vi "RSZVB Get All Calibration Units.vi"(8 "error in (no error)":errorcluster {"code" format="%.0x"}, 11 "VISA session":refnum<visa-resource-name>) -> (0 "error out":errorcluster {"code" format="%.0x"}, 2 "Calibration Unit":string, 3 "dup VISA session":refnum<visa-resource-name>)   [LabVIEW 2011]
doc: "This VI returns the type and address of all calibration units connected to the VNA. \n\nRemote-control command(s):\n:SYSTem:COMMunicate:RDEVice:AKAL:ADDRess:ALL?"
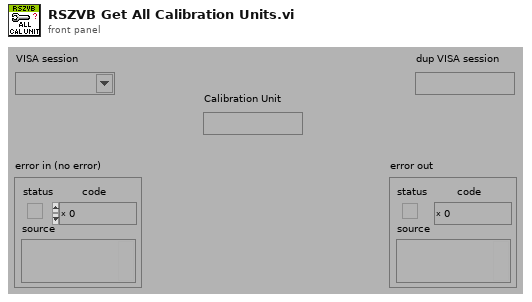
[diagram p1: front panel]
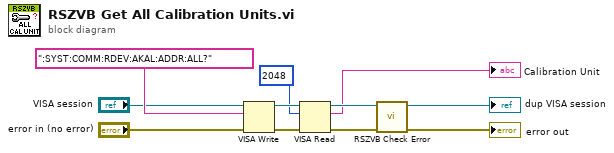
[diagram p0: block diagram]
diagram:
  n1 = VISA Write(VISA resource name="VISA session", write buffer=":SYST:COMM:RDEV:AKAL:ADDR:ALL?" ("format string"), error in (no error)="error in (no error)") -> (VISA resource name out=w10:refnum<visa-resource-name>, error out=w9:errorcluster)  [unwired: 1 out]
  n2 = VISA Read(VISA resource name=w10, byte count=u32 2048 ("byte count (0)"), error in (no error)=w9) -> (VISA resource name out=w7:refnum<visa-resource-name>, read buffer=→"Calibration Unit":string, error out=w6:errorcluster)  [unwired: 1 out]
  n3 = call "RSZVB Check Error.vi"("error in (no error)"=w6, "VISA session"=w7) -> ("error out"=→"error out":errorcluster, "dup VISA session"=→"dup VISA session":refnum<visa-resource-name>)  [unwired: 8 in]
